vi "Pneumatic Control Loop Test.vi"() -> ()   [LabVIEW 2013]
panel:
  out "Finished":bool
  out "Release":bool
  out "Add":bool
  in  "reinit":bool
  in  "Process Variable":dbl(slide) scale=0.0..60.0
  in  "Setpoint":dbl
  in  "stop":bool
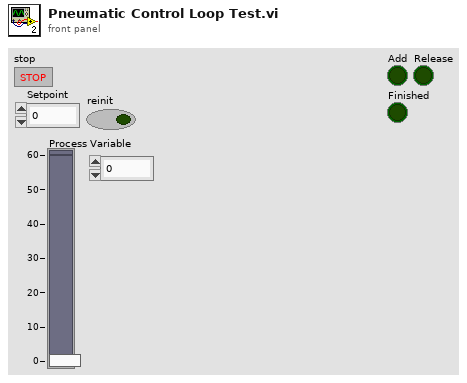
[diagram p1: front panel]
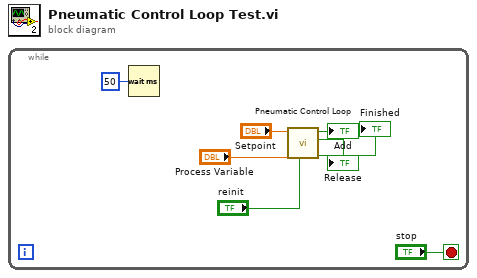
[diagram p0: block diagram]
diagram:
  n1 = while {
    stop <- "stop" stop-if-true
    n2 = Wait (ms)(milliseconds to wait=u32 50) -> ()  [unwired: 1 out]
    n3 = call "Pneumatic Control Loop.vi"("reinit"="reinit", "Process Variable"="Process Variable", "Setpoint"="Setpoint") -> ("Finished"=→"Finished":bool, "Release"=→"Release":bool, "Add"=→"Add":bool)  [unwired: 6 in]
  }
